vi "ziClose.vi"(3 "Error In":errorcluster, 5 "Handle In":T1 {"Handle" format="0x%08x"; "Conn" format="0x%08x"}) -> (0 "Error Out":errorcluster, 2 "Handle Out":T1 {"Handle" format="0x%08x"; "Conn" format="0x%08x"})   [LabVIEW 2009, in "Zurich Instruments LabOne.lvlib"]
doc: "Disconnects from a ziServer and frees resources. Use this vi to terminate a connection."
uses:
  <instrlib>/Zurich Instruments LabOne/Zurich Instruments LabOne.lvlib
  <instrlib>/Zurich Instruments LabOne/Public/ziTypeHandle.ctl
  <instrlib>/Zurich Instruments LabOne/Private/ziLV32.dll
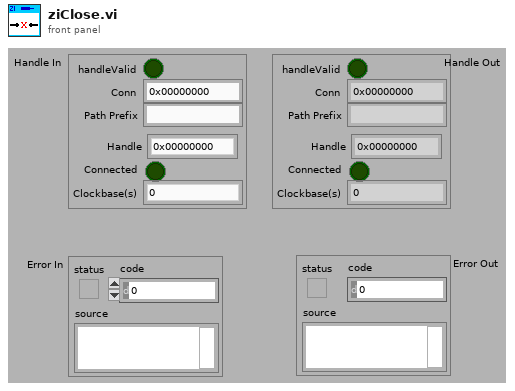
[diagram p1: front panel]
types:
  T1 = typedef "Zurich Instruments LabOne.lvlib/ziTypeHandle.ctl" = cluster{"handleValid":bool, "Conn":u64, "Path Prefix":string, "Handle":u64, "Connected":bool, "Clockbase(s)":dbl}
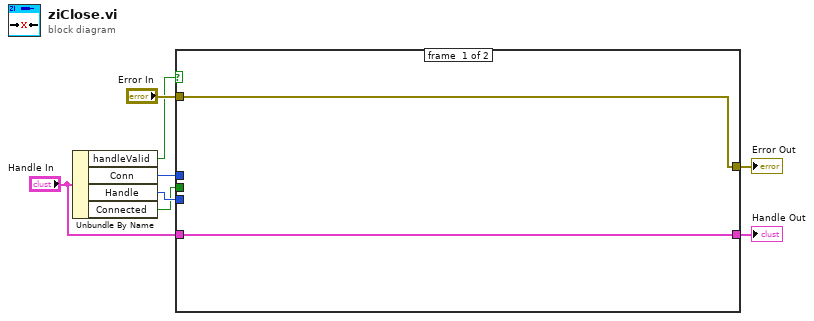
[diagram p0: block diagram]
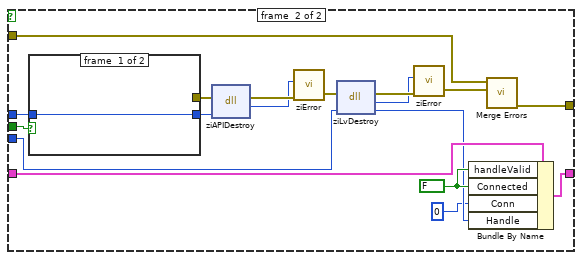
[diagram p2: hidden frame]
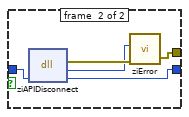
[diagram p3: hidden frame]
diagram:
  n1 = Unbundle By Name("Handle In") -> ("handleValid"=w2:bool, "Conn"=w4:u64, "Handle"=w3:u64, "Connected"=w1:bool)
  n2 = case shown="True" w2 {
    tunnel: w4 -> [_ w28]
    tunnel: "Handle In" -> [w10 w27]
    tunnel: [w10 w26] -> w7
    tunnel: "Error In" -> [w9 w14]
    tunnel: [w9 w12] -> w6
    tunnel: w3 -> [_ w23]
    tunnel: w1 -> [_ w15]
    frame #0 {
    }
    frame #1 {
      w24 = FALSE ("handleOK")
      n3 = case shown="True" w15 {
        tunnel: w28 -> [w29 w34]
        tunnel: [w29 w33] -> w25
        tunnel: [_ w30] -> w11
        frame #0 {
        }
        frame #1 {
          n4 = dll-call lib="C:/Program Files (x86)/National Instruments/LabVIEW 2009/instr.lib/Zurich Instruments LabOne/Private/ziLV*.*" fn="ziAPIDisconnect"("Connection"=w34) -> (error out=w32:errorcluster, "return type"=w31:u32, "Connection"=w33:u64)  [unwired: 3 in, 1 out]
          n5 = call <instrlib>:"ziError.vi"("ziErrorCode"=w31, "Error In"=w32) -> ("Error Out"=w30:errorcluster)  [unwired: 4 in]
        }
      }
      n6 = dll-call lib="C:/Program Files (x86)/National Instruments/LabVIEW 2009/instr.lib/Zurich Instruments LabOne/Private/ziLV*.*" fn="ziAPIDestroy"(error in=w11, "Connection"=w25) -> (error out=w18:errorcluster, "return type"=w16:u32)  [unwired: 3 in, 1 out]
      n7 = call <instrlib>:"ziError.vi"("ziErrorCode"=w16, "Error In"=w18) -> ("Error Out"=w19:errorcluster)  [unwired: 4 in]
      n8 = dll-call lib="C:/Program Files (x86)/National Instruments/LabVIEW 2009/instr.lib/Zurich Instruments LabOne/Private/ziLV*.*" fn="ziLvDestroy" label="ziLVDestroy"(error in=w19, "Handle"=w23) -> (error out=w20:errorcluster, "return type"=w17:u32, "Handle"=w22:u64)  [unwired: 2 in, 1 out]
      n9 = call <instrlib>:"ziError.vi"("ziErrorCode"=w17, "Error In"=w20) -> ("Error Out"=w13:errorcluster)  [unwired: 4 in]
      n10 = Bundle By Name(cluster=w27, "handleValid"=w24, "Connected"=w24, "Conn"=u64 0, "Handle"=w22) -> (w26:T1)
      n11 = call <vilib>:"Merge Errors.vi"("error in 2 (no error)"=w13, "error in 1 (no error)"=w14) -> ("error out"=w12:errorcluster)  [unwired: 5 in]
    }
  }
  "Handle Out" <- w7
  "Error Out" <- w6
